vi "HEWH Panel Communication Settings.vi"(11 "error in (no error)":errorcluster) -> (6 "GEA2 HyperData Out":bool, 15 "error out":errorcluster)   [LabVIEW 2019]
uses:
  Utility/Custom Pallet Controls/Custom Pallet Forward.ctl
panel:
  in  "Combo Box":string(combo)
  out "Description 2":string="GEA2: Uses HEWH Electronic Board for heat source\nstatus updates\n\nNon-GEA2:\nCompressor and Fan = 0.5-5 Amps\nUpper Element - Uses sensing cable\nLower Element - Uses sensing cable\n"
  out "Description":string="Communication Setting"
  in  "Complete":T1
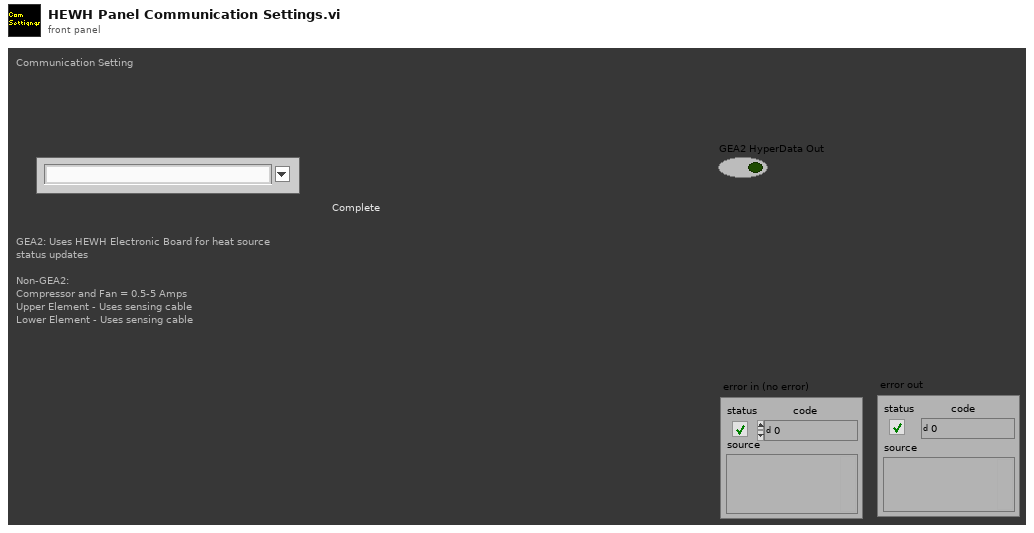
[diagram p1: front panel]
types:
  T1 = typedef "Custom Pallet Forward.ctl" = bool
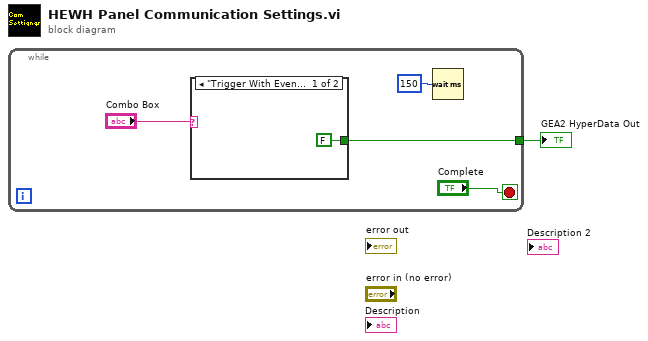
[diagram p0: block diagram]
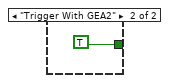
[diagram p2: hidden frame]
diagram:
  n1 = while {
    tunnel: [w2] -> w1
    stop <- "Complete" stop-if-true
    n2 = case shown="\"Trigger With Event Leads\", Default" "Combo Box" {
      tunnel: [FALSE TRUE] -> w2
      frame "Trigger With Event Leads", Default {
      }
      frame "Trigger With GEA2" {
      }
    }
    n3 = Wait (ms)(milliseconds to wait=u32 150) -> ()  [unwired: 1 out]
  }
  "GEA2 HyperData Out" <- w1
